vi "BarLIV_SearchAndPlot_Main_v2.vi"() -> ()   [LabVIEW 2017]
uses:
  <vilib>/Utility/NIReport.llb/NI_report.lvclass
panel:
  in  "DB Table Name":string="Bar_LIV"
  in  "Date Selection":i32[](listbox)
  out "Input selection subarray":string[][](array[string])
  out "Selected Wafer ID":string[](array[string])
  out "Selected Bar WO":string[](array[string])
  out "Selected Bar SN":string[](array[string])
  out "Selected Test Date":string[](array[string])
  out "Input selection Items":string[][](array[string])
  in  "Tab Control":enum32{"Raw Data", "Selected Data"}(tab)
  out "Raw Bar Table Data":string[][](array[string])=[["1", "3/22/2019", "30101152", "DM17-20                  ", "                         ", "31 emitters/Pass", "30", "0.06", "1.375", "933.884", "37.774", "0.145"], ["2", "3/22/2019", "30101152", "DM17-20                  ", "                         ", "31 emitters/Pass", "60", "24.48", "1.414", "935.13", "41.871", "28.854"], ["3", "3/22/2019", "30101152", "DM17-20                  ", "                         ", "31 emitters/Pass", "90", "57.61", "1.445", "935.9", "44.404", "44.298"], ["4", "3/22/2019", "30101152", "DM17-20                  ", "                         ", "31 emitters/Pass", "120", "91.3", "1.475", "936.78", "47.298", "51.582"], ["5", "3/22/2019", "30101152", "DM17-20                  ", "                         ", "31 emitters/Pass", "150", "125", "1.504", "937.76", "50.522", "55.408"], ["6", "3/22/2019", "30101152", "DM17-20                  ", "                         ", "31 emitters/Pass", "180", "158.3", "1.532", "938.84", "54.075", "57.405"], ["7", "3/22/2019", "30101152", "DM17-20                  ", "                         ", "31 emitters/Pass", "210", "191.3", "1.56", "939.97", "57.792", "58.394"], ["8", "3/22/2019", "30101152", "DM17-20                  ", "                         ", "31 emitters/Pass", "240", "222.8", "1.587", "941.25", "62.002", "58.496"], ["9", "3/22/2019", "30101152", "DM17-20                  ", "                         ", "31 emitters/Pass", "270", "253.6", "1.613", "942.63", "66.542", "58.231"], ["10", "3/22/2019", "30101152", "DM17-20                  ", "                         ", "31 emitters/Pass", "300", "282.9", "1.639", "944.11", "71.41", "57.535"], ["11", "3/22/2019", "30101152", "DM17-20                  ", "                         ", "31 emitters/Pass", "330", "311.2", "1.664", "945.73", "76.739", "56.672"], ["12", "3/22/2019", "30101562", "DM17-20                  ", "                         ", "Pass", "30", "0.18", "1.374", "934.413", "37.888", "0.437"], ["13", "3/22/2019", "30101562", "DM17-20                  ", "                         ", "Pass", "60", "25.92", "1.413", "935.59", "41.76", "30.573"], ["14", "3/22/2019", "30101562", "DM17-20                  ", "                         ", "Pass", "90", "59.94", "1.443", "936.37", "44.326", "46.154"], ["15", "3/22/2019", "30101562", "DM17-20                  ", "                         ", "Pass", "120", "94.3", "1.473", "937.19", "47.023", "53.349"], ["16", "3/22/2019", "30101562", "DM17-20                  ", "                         ", "Pass", "150", "128.7", "1.502", "938.12", "50.083", "57.124"], ["17", "3/22/2019", "30101562", "DM17-20                  ", "                         ", "Pass", "180", "162.8", "1.53", "939.14", "53.438", "59.114"], ["18", "3/22/2019", "30101562", "DM17-20                  ", "                         ", "Pass", "210", "196.5", "1.557", "940.27", "57.155", "60.097"], ["19", "3/22/2019", "30101562", "DM17-20                  ", "                         ", "Pass", "240", "229.2", "1.584", "941.5", "61.201", "60.29"], ["20", "3/22/2019", "30101562", "DM17-20                  ", "                         ", "Pass", "270", "261", "1.61", "942.83", "65.576", "60.041"], ["21", "3/22/2019", "30101562", "DM17-20                  ", "                         ", "Pass", "300", "291.7", "1.635", "944.21", "70.115", "59.47"], ["22", "3/22/2019", "30101562", "DM17-20                  ", "                         ", "Pass", "330", "320.8", "1.659", "945.83", "75.444", "58.597"], ["23", "3/22/2019", "30101566", "DM17-20                  ", "                         ", "Fail", "30", "0.14", "1.375", "934.203", "37.774", "0.339"], ["24", "3/22/2019", "30101566", "DM17-20                  ", "                         ", "Fail", "60", "25.11", "1.413", "935.39", "41.68", "29.618"], ["25", "3/22/2019", "30101566", "DM17-20                  ", "                         ", "Fail", "90", "58.98", "1.444", "936.11", "44.048", "45.383"], ["26", "3/22/2019", "30101566", "DM17-20                  ", "                         ", "Fail", "120", "93.3", "1.473", "936.93", "46.745", "52.783"], ["27", "3/22/2019", "30101566", "DM17-20                  ", "                         ", "Fail", "150", "127.7", "1.502", "937.91", "49.969", "56.68"], ["28", "3/22/2019", "30101566", "DM17-20                  ", "                         ", "Fail", "180", "161.8", "1.53", "938.84", "53.028", "58.751"], ["29", "3/22/2019", "30101566", "DM17-20                  ", "                         ", "Fail", "210", "195.3", "1.558", "939.97", "56.745", "59.692"], ["30", "3/22/2019", "30101566", "DM17-20                  ", "                         ", "Fail", "240", "228.2", "1.584", "941.04", "60.265", "60.027"], ["31", "3/22/2019", "30101566", "DM17-20                  ", "                         ", "Fail", "270", "260.1", "1.61", "942.37", "64.64", "59.834"], ["32", "3/22/2019", "30101566", "DM17-20                  ", "                         ", "Fail", "300", "290.9", "1.635", "943.75", "69.18", "59.307"], ["33", "3/22/2019", "30101566", "DM17-20                  ", "                         ", "Fail", "330", "320.2", "1.66", "945.28", "74.212", "58.452"], ["34", "3/22/2019", "30101586", "DM17-20                  ", "                         ", "Pass", "30", "0.12", "1.375", "934.057", "37.55", "0.291"], ["35", "3/22/2019", "30101586", "DM17-20                  ", "                         ", "Pass", "60", "24.93", "1.415", "935.23", "41.41", "29.364"], ["36", "3/22/2019", "30101586", "DM17-20                  ", "                         ", "Pass", "90", "58.6", "1.447", "935.95", "43.778", "44.997"], ["37", "3/22/2019", "30101586", "DM17-20                  ", "                         ", "Pass", "120", "92.9", "1.478", "936.78", "46.509", "52.379"], ["38", "3/22/2019", "30101586", "DM17-20                  ", "                         ", "Pass", "150", "127.3", "1.507", "937.71", "49.568", "56.315"], ["39", "3/22/2019", "30101586", "DM17-20                  ", "                         ", "Pass", "180", "161.3", "1.537", "938.68", "52.759", "58.303"], ["40", "3/22/2019", "30101586", "DM17-20                  ", "                         ", "Pass", "210", "194.7", "1.565", "939.76", "56.311", "59.242"], ["41", "3/22/2019", "30101586", "DM17-20                  ", "                         ", "Pass", "240", "227.6", "1.593", "940.89", "60.028", "59.531"], ["42", "3/22/2019", "30101586", "DM17-20                  ", "                         ", "Pass", "270", "259.4", "1.62", "942.12", "64.075", "59.305"], ["43", "3/22/2019", "30101586", "DM17-20                  ", "                         ", "Pass", "300", "290.1", "1.647", "943.49", "68.581", "58.713"], ["44", "3/22/2019", "30101586", "DM17-20                  ", "                         ", "Pass", "330", "319.4", "1.673", "945.02", "73.614", "57.853"], ["45", "3/22/2019", "30101731", "DM17-20                  ", "                         ", "31 emitters/Pass", "30", "0.18", "1.375", "933.644", "37.885", "0.436"], ["46", "3/22/2019", "30101731", "DM17-20                  ", "                         ", "31 emitters/Pass", "60", "24.92", "1.415", "934.87", "41.92", "29.352"], ["47", "3/22/2019", "30101731", "DM17-20                  ", "                         ", "31 emitters/Pass", "90", "58.52", "1.446", "935.64", "44.453", "44.967"], ["48", "3/22/2019", "30101731", "DM17-20                  ", "                         ", "31 emitters/Pass", "120", "92.7", "1.475", "936.47", "47.183", "52.373"], ["49", "3/22/2019", "30101731", "DM17-20                  ", "                         ", "31 emitters/Pass", "150", "126.8", "1.505", "937.45", "50.407", "56.168"], ["50", "3/22/2019", "30101731", "DM17-20                  ", "                         ", "31 emitters/Pass", "180", "160.3", "1.533", "938.48", "53.795", "58.092"], ["51", "3/22/2019", "30101731", "DM17-20                  ", "                         ", "31 emitters/Pass", "210", "192.9", "1.561", "939.55", "57.314", "58.845"], ["52", "3/22/2019", "30101731", "DM17-20                  ", "                         ", "31 emitters/Pass", "240", "224.9", "1.588", "940.73", "61.196", "59.01"], ["53", "3/22/2019", "30101731", "DM17-20                  ", "                         ", "31 emitters/Pass", "270", "255.6", "1.614", "942.06", "65.571", "58.653"], ["54", "3/22/2019", "30101731", "DM17-20                  ", "                         ", "31 emitters/Pass", "300", "285.6", "1.64", "943.54", "70.439", "58.049"], ["55", "3/22/2019", "30101731", "DM17-20                  ", "                         ", "31 emitters/Pass", "330", "313.9", "1.665", "945.12", "75.637", "57.13"]]
  out "Data Selected (<10)":string[][](array[string])
  in  "Bar SN Selection":i32[](listbox)
  in  "Bar WO Selection":i32[](listbox)
  in  "Wafer ID Selection":i32[](listbox)=[0]
  out "BarWO Select Output Subarry":string[][](array[string])=[["03/22/2019", "201", "1", "1"], ["03/22/2019", "201", "1", "2"], ["03/22/2019", "204", "3", "2"]]
  out "WaferID Select Output Subarry":string[][](array[string])=[["03/22/2019", "201", "1", "1"], ["03/22/2019", "201", "1", "2"], ["03/22/2019", "204", "2", "1"], ["03/22/2019", "204", "3", "2"], ["03/22/2018", "205", "4", ""], ["03/22/2018", "206", "5", ""], ["03/22/2018", "207", "7", ""], ["03/22/2018", "208", "7", ""]]
  in  "Stop and Plot":bool
  in  "Input File Name":string="BarLIV"
  in  "File Directory to Save Report":path=path "H:/PT_Projects/DM17/57_Testing/DM17_report/20190611_BarLIV_DB_Installation/DataReport_Template/Report_output"
  in  "Report Template":path=path "H:/PT_Projects/DM17/57_Testing/DM17_report/20190611_BarLIV_DB_Installation/DataReport_Template/Bar_LIV_ExcelTemp.xlsx"
  out "Select Data":string[][](array[string])=[["23", "3/22/2019", "30101566", "DM17-20                  ", "                         ", "Fail", "30", "0.14", "1.375", "934.203", "37.774", "0.339"], ["24", "3/22/2019", "30101566", "DM17-20                  ", "                         ", "Fail", "60", "25.11", "1.413", "935.39", "41.68", "29.618"], ["25", "3/22/2019", "30101566", "DM17-20                  ", "                         ", "Fail", "90", "58.98", "1.444", "936.11", "44.048", "45.383"], ["26", "3/22/2019", "30101566", "DM17-20                  ", "                         ", "Fail", "120", "93.3", "1.473", "936.93", "46.745", "52.783"], ["27", "3/22/2019", "30101566", "DM17-20                  ", "                         ", "Fail", "150", "127.7", "1.502", "937.91", "49.969", "56.68"], ["28", "3/22/2019", "30101566", "DM17-20                  ", "                         ", "Fail", "180", "161.8", "1.53", "938.84", "53.028", "58.751"], ["29", "3/22/2019", "30101566", "DM17-20                  ", "                         ", "Fail", "210", "195.3", "1.558", "939.97", "56.745", "59.692"], ["30", "3/22/2019", "30101566", "DM17-20                  ", "                         ", "Fail", "240", "228.2", "1.584", "941.04", "60.265", "60.027"], ["31", "3/22/2019", "30101566", "DM17-20                  ", "                         ", "Fail", "270", "260.1", "1.61", "942.37", "64.64", "59.834"], ["32", "3/22/2019", "30101566", "DM17-20                  ", "                         ", "Fail", "300", "290.9", "1.635", "943.75", "69.18", "59.307"], ["33", "3/22/2019", "30101566", "DM17-20                  ", "                         ", "Fail", "330", "320.2", "1.66", "945.28", "74.212", "58.452"]]
  in  "Finish Selection":bool
  out "Error Out":errorcluster
  in  "Error In":errorcluster
  # "Bar LIV Selection From RD Database - Chao Gong"
  # "Step: \n1) Input database name and select report template.\n2) Input report saving direcotry. Name the ouput report.\n1) Select wafer ID, Bar WO, Bar SN and Date in sequence. (All for all selection). \n2) Click finish selection.\n3) Click stop to generate and save plotting report\n4) No more 10 selection a time (Excel template runs out)"
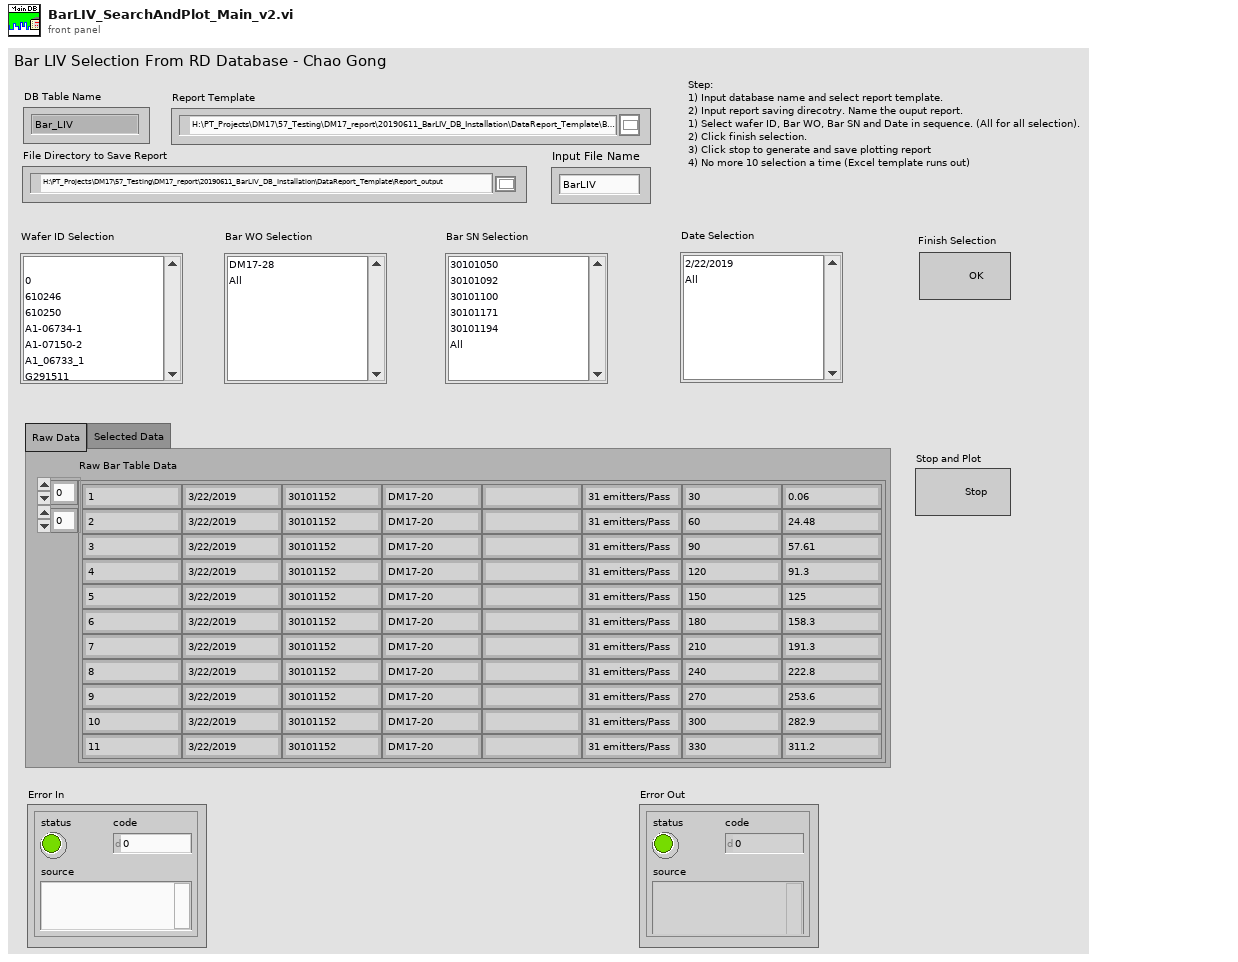
[diagram p1: front panel]
types:
  T1 = enum16{"Standard Report", "HTML", "Word", "Excel"}
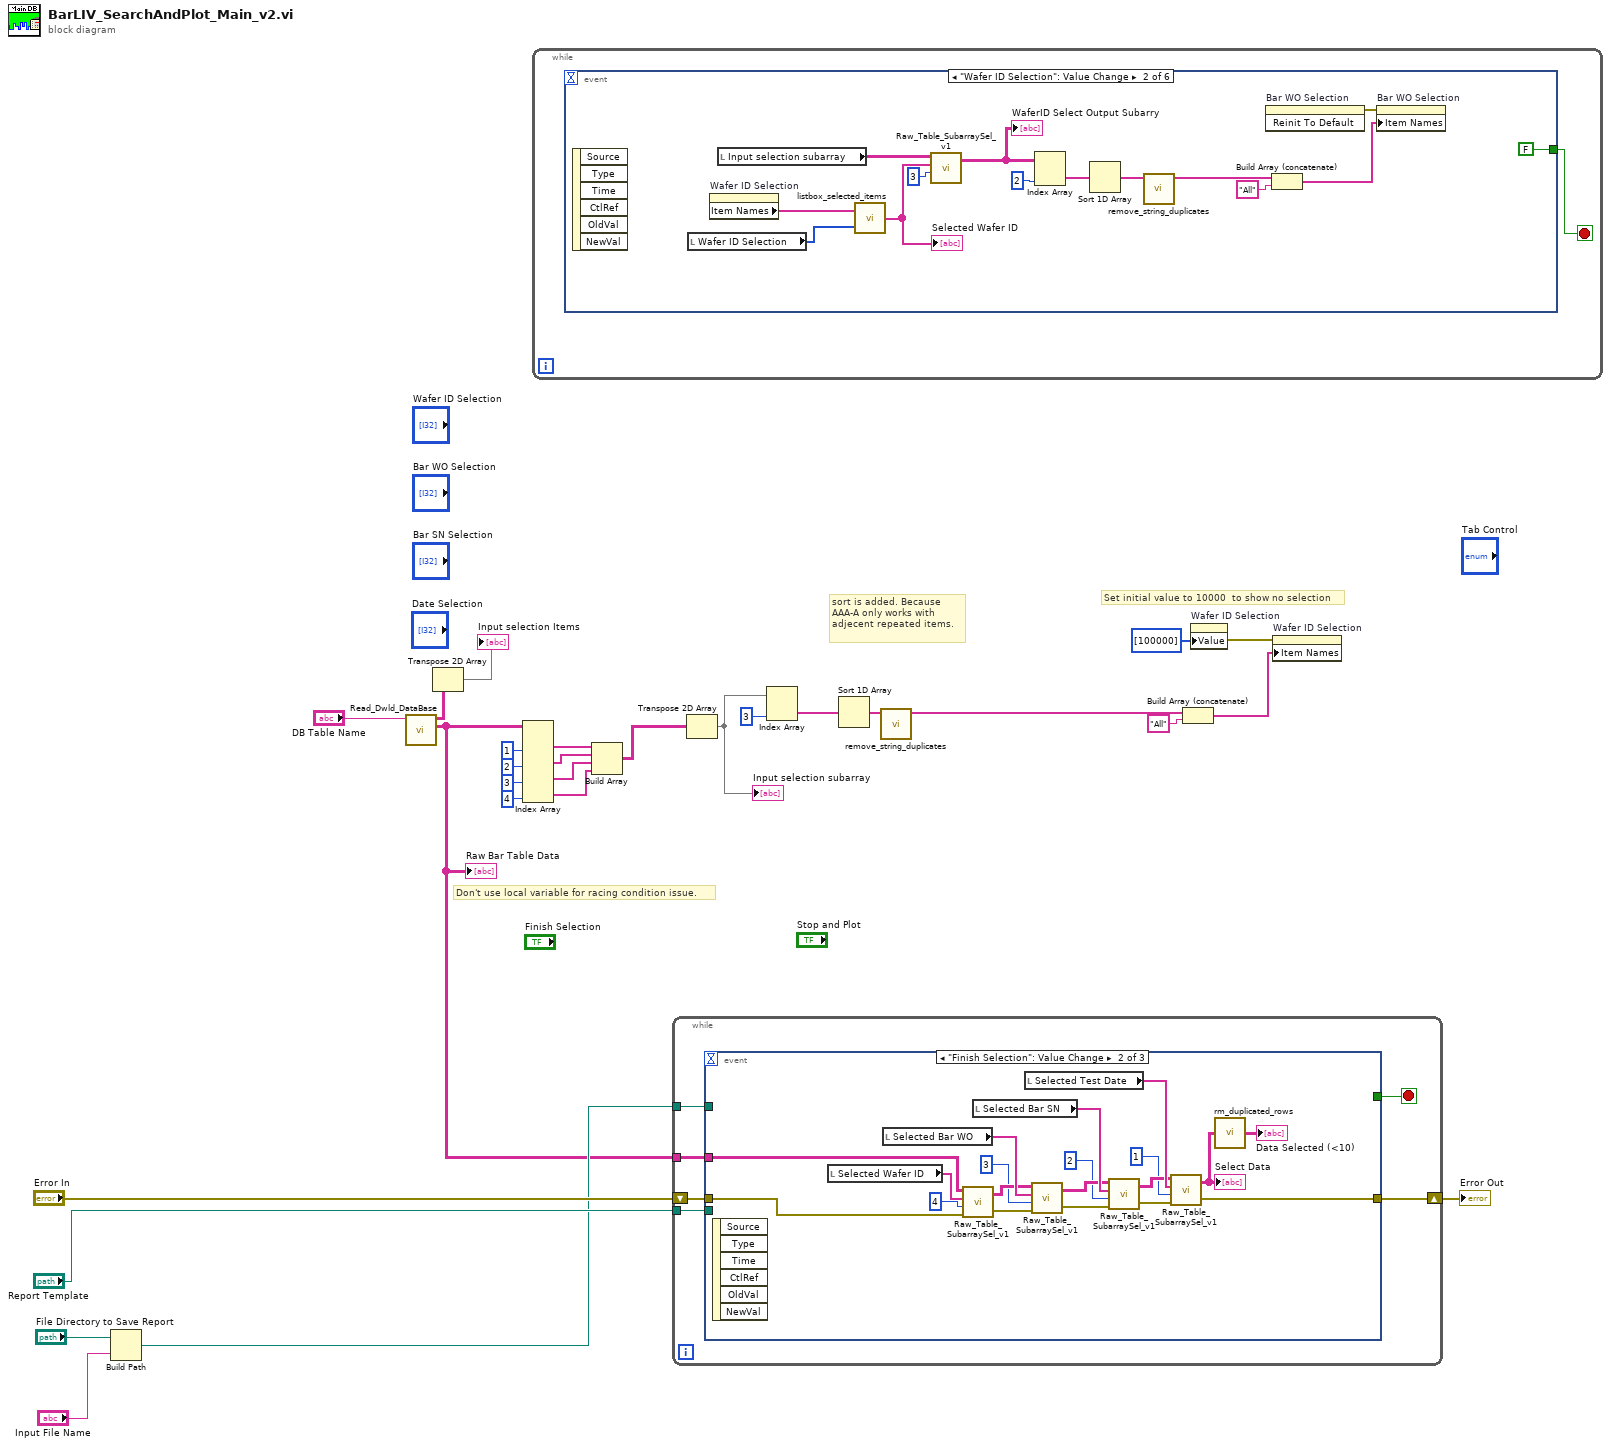
[diagram p0: block diagram]
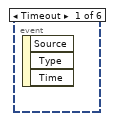
[diagram p2: hidden frame]
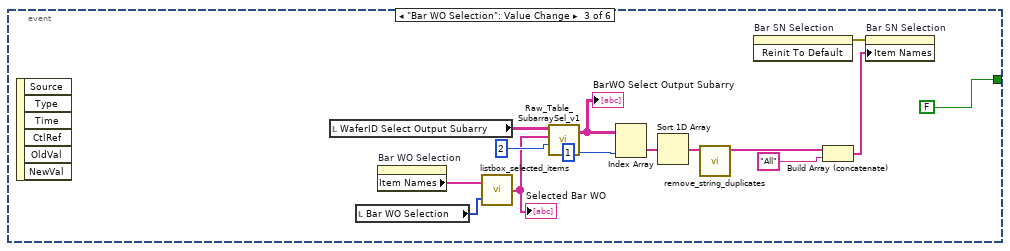
[diagram p3: hidden frame]
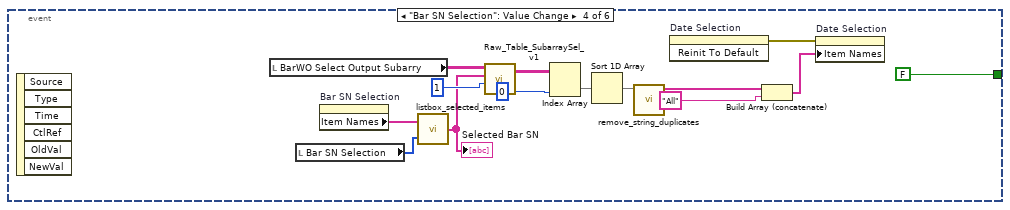
[diagram p4: hidden frame]
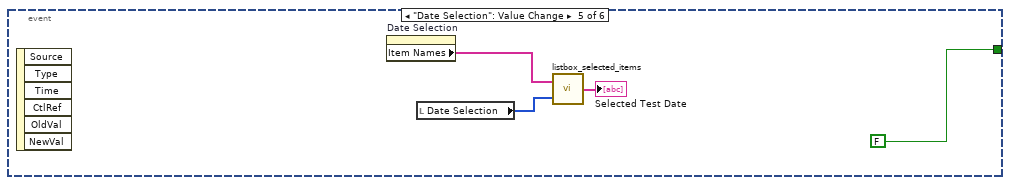
[diagram p5: hidden frame]
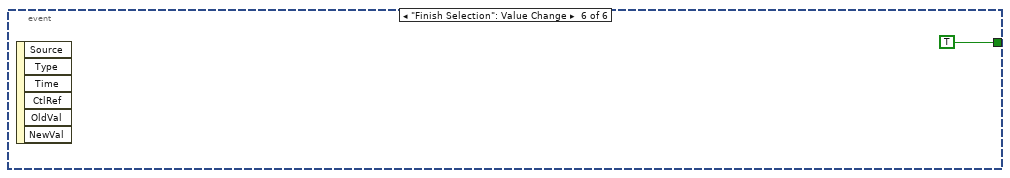
[diagram p6: hidden frame]
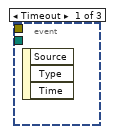
[diagram p7: hidden frame]
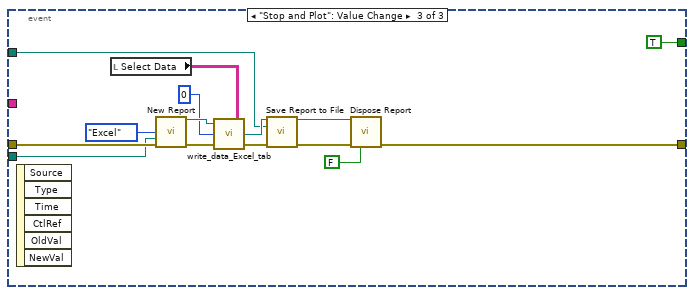
[diagram p8: hidden frame]
diagram:
  # "Don't use local variable for racing condition issue."
  # "Set initial value to 10000  to show no selection"
  # "sort is added. Because AAA-A only works with adjecent repeated items."
  n1 = Build Path(base path="File Directory to Save Report", name or relative path="Input File Name") -> (appended path=w24:path)
  n2 = call "Read_Dwld_DataBase.vi"("Select Table Name"="DB Table Name") -> ("Output Data"=w1:string[][], "Output selection string"=w18:string[][])  [unwired: 3 in, 2 out]
  "Raw Bar Table Data" <- w1
  n3 = Transpose 2D Array(2D array=w18) -> (transposed array=→"Input selection Items":string[][])
  n4 = Index Array(array=w1, index (col) #1=1 ("disabled index (col)"), index (col) #2=2 ("index (col)"), index (col) #3=3 ("index (col)"), index (col) #4=4 ("index (col)")) -> (element #1=w12:string[], element #2=w11:string[], element #3=w10:string[], element #4=w9:string[])  [unwired: 4 in]
  n5 = while {
    stop <- w29 stop-if-true
    n6 = event shown="[1] \"Wafer ID Selection\": Value Change" {
      selector: _ -> [_ _ _ _ _ _]
      dyn-events: _ -> [_ _ _ _ _ _]
      timeout: _ -> [_ _ _ _ _ _]
      tunnel: [_ FALSE ("stop") FALSE ("stop") FALSE ("stop") FALSE ("stop") TRUE ("stop")] -> w29
      event Timeout {
        n7 = event-data() -> ()  [unwired: 1 in, 3 out]
      }
      event "Wafer ID Selection": Value Change {
        n8 = event-data() -> ()  [unwired: 1 in, 6 out]
        n9 = local read "Wafer ID Selection"() -> (w34:i32[])
        n10 = property on="Wafer ID Selection" class="LstBox (strict)"() -> ("Item Names"=w35:string[])  [unwired: 2 in, 2 out]
        n11 = local read "Input selection subarray"() -> (w43:string[][])
        n12 = call "listbox_selected_items.vi"("Selected item number"=w34, "All items"=w35) -> ("Selected items"=w33:string[])
        "Selected Wafer ID" <- w33
        n13 = call "Raw_Table_SubarraySel_v1.vi"("Column Index"=3, "String to compare"=w33, "Raw Bar Table Data"=w43) -> ("Selected Output"=w40:string[][])  [unwired: 1 in, 1 out]
        "WaferID Select Output Subarry" <- w40
        n14 = Index Array(array=w40, index (col)=2 ("disabled index (col)")) -> (element=w32:string[])  [unwired: 1 in]
        n15 = Sort 1D Array(array=w32) -> (sorted array=w31:string[])
        n16 = call "remove_string_duplicates.vi"("In"=w31) -> ("Out"=w30:string[])  [unwired: 10 in]
        n17 = invoke on="Bar WO Selection" class="LstBox (strict)" method="Reinit To Default"() -> (error out=w36:errorcluster)  [unwired: 3 in, 2 out]
        n18 = Build Array (concatenate)(w30, "All") -> (w37:string[])
        n19 = property on="Bar WO Selection" class="LstBox (strict)"(error in=w36, "Item Names"=w37) -> ()  [unwired: 1 in, 2 out]
      }
      event "Bar WO Selection": Value Change {
        n20 = event-data() -> ()  [unwired: 1 in, 6 out]
        n21 = local read "WaferID Select Output Subarry"() -> (w57:string[][])
        n22 = local read "Bar WO Selection"() -> (w48:i32[])
        n23 = property on="Bar WO Selection" class="LstBox (strict)"() -> ("Item Names"=w49:string[])  [unwired: 2 in, 2 out]
        n24 = call "listbox_selected_items.vi"("Selected item number"=w48, "All items"=w49) -> ("Selected items"=w47:string[])
        "Selected Bar WO" <- w47
        n25 = call "Raw_Table_SubarraySel_v1.vi"("Column Index"=2, "String to compare"=w47, "Raw Bar Table Data"=w57) -> ("Selected Output"=w55:string[][])  [unwired: 1 in, 1 out]
        "BarWO Select Output Subarry" <- w55
        n26 = Index Array(array=w55, index (col)=1 ("disabled index (col)")) -> (element=w46:string[])  [unwired: 1 in]
        n27 = Sort 1D Array(array=w46) -> (sorted array=w45:string[])
        n28 = call "remove_string_duplicates.vi"("In"=w45) -> ("Out"=w44:string[])  [unwired: 10 in]
        n29 = invoke on="Bar SN Selection" class="LstBox (strict)" method="Reinit To Default"() -> (error out=w50:errorcluster)  [unwired: 3 in, 2 out]
        n30 = Build Array (concatenate)(w44, "All") -> (w51:string[])
        n31 = property on="Bar SN Selection" class="LstBox (strict)"(error in=w50, "Item Names"=w51) -> ()  [unwired: 1 in, 2 out]
      }
      event "Bar SN Selection": Value Change {
        n32 = event-data() -> ()  [unwired: 1 in, 6 out]
        n33 = local read "BarWO Select Output Subarry"() -> (w71:string[][])
        n34 = local read "Bar SN Selection"() -> (w64:i32[])
        n35 = property on="Bar SN Selection" class="LstBox (strict)"() -> ("Item Names"=w65:string[])  [unwired: 2 in, 2 out]
        n36 = call "listbox_selected_items.vi"("Selected item number"=w64, "All items"=w65) -> ("Selected items"=w63:string[])
        "Selected Bar SN" <- w63
        n37 = call "Raw_Table_SubarraySel_v1.vi"("Column Index"=1, "String to compare"=w63, "Raw Bar Table Data"=w71) -> ("Selected Output"=w69:string[][])  [unwired: 1 in, 1 out]
        n38 = Index Array(array=w69, index (col)=0 ("disabled index (col)")) -> (element=w62:string[])  [unwired: 1 in]
        n39 = Sort 1D Array(array=w62) -> (sorted array=w61:string[])
        n40 = call "remove_string_duplicates.vi"("In"=w61) -> ("Out"=w58:string[])  [unwired: 10 in]
        n41 = invoke on="Date Selection" class="LstBox (strict)" method="Reinit To Default"() -> (error out=w59:errorcluster)  [unwired: 3 in, 2 out]
        n42 = Build Array (concatenate)(w58, "All") -> (w60:string[])
        n43 = property on="Date Selection" class="LstBox (strict)"(error in=w59, "Item Names"=w60) -> ()  [unwired: 1 in, 2 out]
      }
      event "Date Selection": Value Change {
        n44 = event-data() -> ()  [unwired: 1 in, 6 out]
        n45 = property on="Date Selection" class="LstBox (strict)"() -> ("Item Names"=w73:string[])  [unwired: 2 in, 2 out]
        n46 = local read "Date Selection"() -> (w75:i32[])
        n47 = call "listbox_selected_items.vi"("Selected item number"=w75, "All items"=w73) -> ("Selected items"=→"Selected Test Date":string[])
      }
      event "Finish Selection": Value Change {
        n48 = event-data() -> ()  [unwired: 1 in, 6 out]
      }
    }
  }
  n49 = Build Array(w12, w11, w10, w9) -> (w8:string[][])
  n50 = while {
    tunnel: w1 -> [w82]
    shift-right: [w80] -> w27
    shift-left: "Error In" -> [w81]
    tunnel: "Report Template" -> [w79]
    tunnel: w24 -> [w78]
    stop <- w77 stop-if-true
    n51 = event shown="[1] \"Finish Selection\": Value Change" {
      selector: _ -> [_ _ _]
      dyn-events: _ -> [_ _ _]
      timeout: _ -> [_ _ _]
      tunnel: w82 -> [_ w85 _]
      tunnel: w81 -> [_ w90 w114]
      tunnel: [_ w86 w109] -> w80
      tunnel: w79 -> [_ _ w112]
      tunnel: w78 -> [_ _ w106]
      tunnel: [_ _ TRUE ("Stop Search and Plot")] -> w77
      event Timeout {
        n52 = event-data() -> ()  [unwired: 1 in, 3 out]
      }
      event "Finish Selection": Value Change {
        n53 = event-data() -> ()  [unwired: 1 in, 6 out]
        n54 = local read "Selected Wafer ID"() -> (w101:string[])
        n55 = local read "Selected Bar WO"() -> (w99:string[])
        n56 = call "Raw_Table_SubarraySel_v1.vi"("error in (no error)"=w90, "Column Index"=4, "String to compare"=w101, "Raw Bar Table Data"=w85) -> ("error out"=w89:errorcluster, "Selected Output"=w98:string[][])
        n57 = local read "Selected Bar SN"() -> (w96:string[])
        n58 = local read "Selected Test Date"() -> (w93:string[])
        n59 = call "Raw_Table_SubarraySel_v1.vi"("error in (no error)"=w89, "Column Index"=3, "String to compare"=w99, "Raw Bar Table Data"=w98) -> ("error out"=w88:errorcluster, "Selected Output"=w95:string[][])
        n60 = call "Raw_Table_SubarraySel_v1.vi"("error in (no error)"=w88, "Column Index"=2, "String to compare"=w96, "Raw Bar Table Data"=w95) -> ("error out"=w87:errorcluster, "Selected Output"=w92:string[][])
        n61 = call "Raw_Table_SubarraySel_v1.vi"("error in (no error)"=w87, "Column Index"=1, "String to compare"=w93, "Raw Bar Table Data"=w92) -> ("error out"=w86:errorcluster, "Selected Output"=w84:string[][])
        "Select Data" <- w84
        n62 = call "rm_duplicated_rows.vi"("Select Data"=w84) -> ("Output Data"=→"Data Selected (<10)":string[][])
      }
      event "Stop and Plot": Value Change {
        n63 = event-data() -> ()  [unwired: 1 in, 6 out]
        n64 = local read "Select Data"() -> (w116:string[][])
        n65 = call <vilib>:"New Report.vi"("report type"=T1."Excel", "template (empty)"=w112, "error in (no error)"=w114) -> ("report out"=w115:refnum<class "NI_report.lvclass">, "error out"=w113:errorcluster)  [unwired: 3 in, 8 out]
        n66 = call "write_data_Excel_tab.vi"("text data"=w116, "error in (no error)"=w113, "worksheet index (0)"=0, "report in"=w115) -> ("error out"=w105:errorcluster, "report out"=w107:refnum<class "NI_report.lvclass">)
        n67 = call-dynamic "Save Report to File.vi"("report in"=w107, "report file path"=w106, "error in (no error)"=w105) -> ("report out"=w104:refnum<class "NI_report.lvclass">, "error out"=w103:errorcluster)  [unwired: 11 in]
        n68 = call-dynamic "Dispose Report.vi"("report in"=w104, "error in (no error)"=w103, "close report? (T)"=FALSE) -> ("error out"=w109:errorcluster)  [unwired: 12 in]
      }
    }
  }
  "Error Out" <- w27
  n69 = Transpose 2D Array(2D array=w8) -> (transposed array=w7:string[][])
  "Input selection subarray" <- w7
  n70 = Index Array(array=w7, index (col)=3 ("disabled index (col)")) -> (element=w20:string[])  [unwired: 1 in]
  n71 = Sort 1D Array(array=w20) -> (sorted array=w19:string[])
  n72 = call "remove_string_duplicates.vi"("In"=w19) -> ("Out"=w5:string[])  [unwired: 10 in]
  n73 = Build Array (concatenate)(w5, "All") -> (w6:string[])
  n74 = property on="Wafer ID Selection" class="LstBox (strict)"("Value"=i32[] [100000] ("Wafer ID Selection")) -> (error out=w4:errorcluster)  [unwired: 2 in, 1 out]
  n75 = property on="Wafer ID Selection" class="LstBox (strict)"(error in=w4, "Item Names"=w6) -> ()  [unwired: 1 in, 2 out]
